vi "Day 16 Testing Custom Boolean Gates.vi"() -> ()   [LabVIEW 2026]
panel:
  out "NOT Verification Grid":bool[](array[boolean])
  out "OR Verification Grid":bool[][](array[boolean])
  out "AND Verification Grid":bool[][](array[boolean])
  out "0, 3":i16[](array[numeric])
  out "Array":bool[](array[boolean])
  out "0, 2":i16[][](array[numeric])
  out "OR Truth Table Grid":bool[][](array[boolean])
  out "0, 1":i16[][](array[numeric])
  out "Output":bool
  in  "Input":bool
  out "Output Y 2":bool
  out "Output Y":bool
  in  "Input B":bool
  in  "Input A":bool
  in  "Input B 2":bool
  in  "Input A 2":bool
  out "AND Truth Table Grid":bool[][](array[boolean])
  # "CUSTOM AND GATE TESTING"
  # "CUSTOM OR GATE TESTING"
  # "CUSTOM NOT GATE TESTING"
  # "CUSTOM AND GATE TRUTH TABLE AND VERIFICATION GRID"
  # "CUSTOM OR GATE TRUTH TABLE AND VERIFICATION GRID"
  # "CUSTOM NOT GATE TRUTH TABLE AND VERIFICATION GRID"
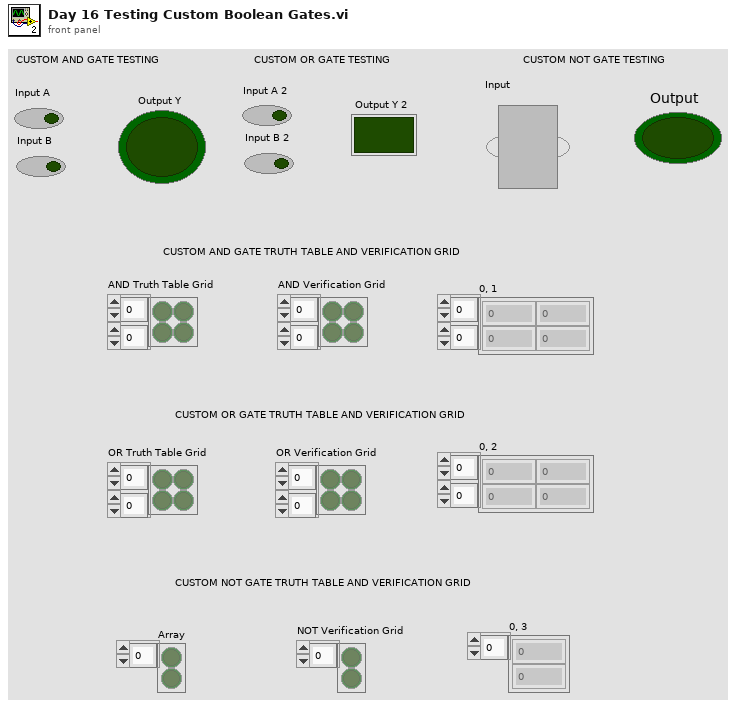
[diagram p1: front panel]
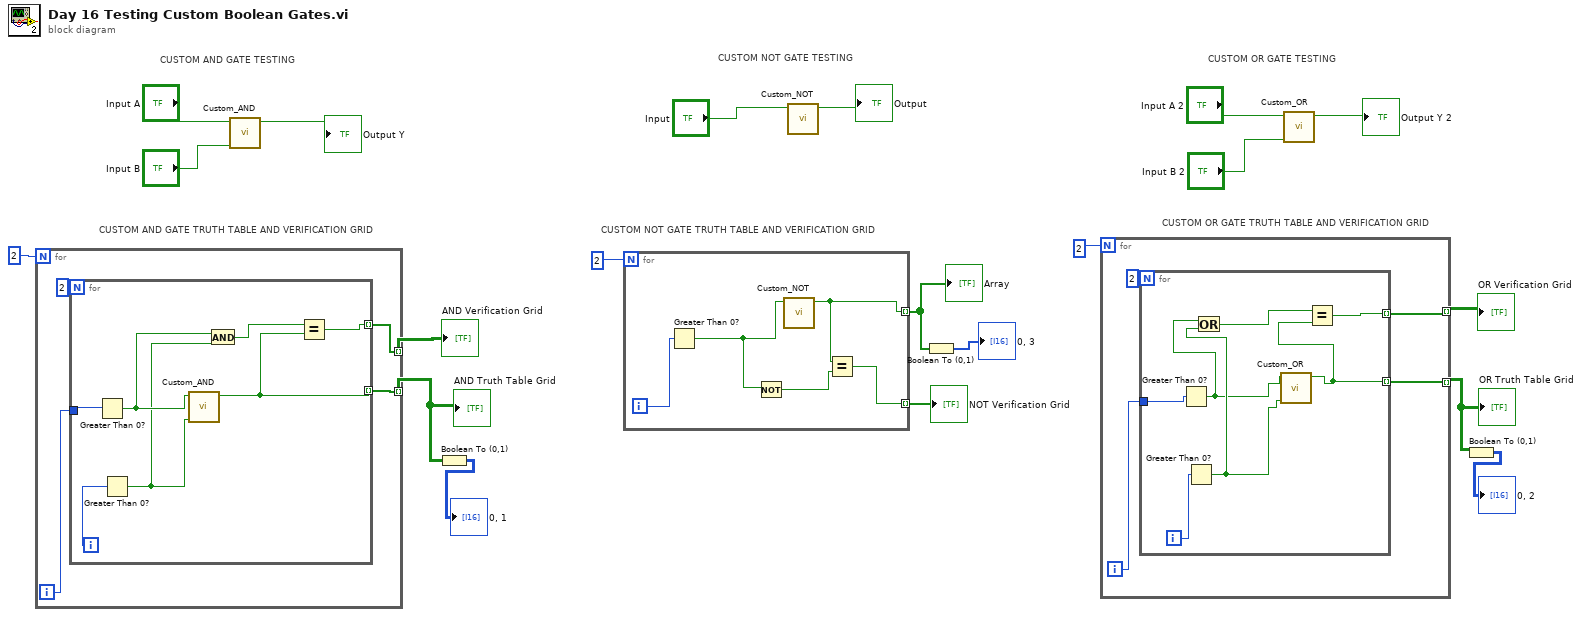
[diagram p0: block diagram]
diagram:
  # "CUSTOM AND GATE TESTING"
  # "CUSTOM NOT GATE TESTING"
  # "CUSTOM OR GATE TESTING"
  # "CUSTOM NOT GATE TRUTH TABLE AND VERIFICATION GRID"
  # "CUSTOM OR GATE TRUTH TABLE AND VERIFICATION GRID"
  # "CUSTOM AND GATE TRUTH TABLE AND VERIFICATION GRID"
  n1 = for {
    N: 2 -> [_]
    tunnel: [w22] -> w11 mode=indexing
    tunnel: [w21] -> w4 mode=indexing
    i -> [w23]
    n2 = for {
      N: 2 -> [_]
      tunnel: w23 -> [w31]
      tunnel: [w26] -> w22 mode=indexing
      tunnel: [w25] -> w21 mode=indexing
      i -> [w30]
      n3 = Greater Than 0?(x=w31) -> (x > 0?=w29:bool)
      n4 = Greater Than 0?(x=w30) -> (x > 0?=w28:bool)
      n5 = call "Custom_AND.vi"("Input B"=w28, "Input A"=w29) -> ("Output Y"=w26:bool)  [unwired: 9 in]
      n6 = And(x=w29, y=w28) -> (x .and. y?=w27:bool)
      n7 = Equal?(x=w27, y=w26) -> (x = y?=w25:bool)
    }
  }
  "AND Truth Table Grid" <- w11
  "AND Verification Grid" <- w4
  n8 = call "Custom_AND.vi"("Input B"="Input B", "Input A"="Input A") -> ("Output Y"=→"Output Y":bool)  [unwired: 9 in]
  n9 = Boolean To (0,1)(Boolean=w11) -> (0, 1=→"0, 1":i16[][])
  n10 = for {
    N: 2 -> [_]
    tunnel: [w34] -> w6 mode=indexing
    tunnel: [w32] -> w2 mode=indexing
    i -> [w36]
    n11 = Greater Than 0?(x=w36) -> (x > 0?=w35:bool)
    n12 = Not(x=w35) -> (.not. x?=w33:bool)
    n13 = call "Custom_NOT.vi"("Input"=w35) -> ("Output"=w34:bool)  [unwired: 10 in]
    n14 = Equal?(x=w34, y=w33) -> (x = y?=w32:bool)
  }
  "Array" <- w6
  "NOT Verification Grid" <- w2
  n15 = call "Custom_NOT.vi"("Input"="Input") -> ("Output"=→"Output":bool)  [unwired: 10 in]
  n16 = Boolean To (0,1)(Boolean=w6) -> (0, 1=→"0, 3":i16[])
  n17 = for {
    N: 2 -> [_]
    tunnel: [w38] -> w9 mode=indexing
    tunnel: [w37] -> w3 mode=indexing
    i -> [w39]
    n18 = for {
      N: 2 -> [_]
      tunnel: w39 -> [w47]
      tunnel: [w43] -> w38 mode=indexing
      tunnel: [w42] -> w37 mode=indexing
      i -> [w46]
      n19 = Greater Than 0?(x=w47) -> (x > 0?=w41:bool)
      n20 = Greater Than 0?(x=w46) -> (x > 0?=w45:bool)
      n21 = Or(x=w41, y=w45) -> (x .or. y?=w44:bool)
      n22 = call "Custom_OR.vi"("Input B"=w45, "Input A"=w41) -> ("Output Y"=w43:bool)  [unwired: 9 in]
      n23 = Equal?(x=w44, y=w43) -> (x = y?=w42:bool)
    }
  }
  "OR Truth Table Grid" <- w9
  "OR Verification Grid" <- w3
  n24 = call "Custom_OR.vi"("Input B"="Input B 2", "Input A"="Input A 2") -> ("Output Y"=→"Output Y 2":bool)  [unwired: 9 in]
  n25 = Boolean To (0,1)(Boolean=w9) -> (0, 1=→"0, 2":i16[][])
